vi "Write Previous State.vi"(8 "error in (no error)":errorcluster, 10 "Previous State":i32[](array[numeric]), 11 "FW Arduino Control in":refnum<class "FW Arduino Control.lvclass">) -> (0 "error out":errorcluster, 3 "FW Arduino Control out":refnum<class "FW Arduino Control.lvclass">)   [LabVIEW 2021, in "FW Arduino Control.lvclass"]
uses:
  FW Arduino Control.lvclass
  C:/Development/prime/Prime-RIMAS/Filter Wheel/Filter Wheel Object/Filter Wheel.lvclass
  Filter Wheel Object/Filter Wheel.lvclass
  FW Arduino Control.lvclass/FW Arduino Control.ctl
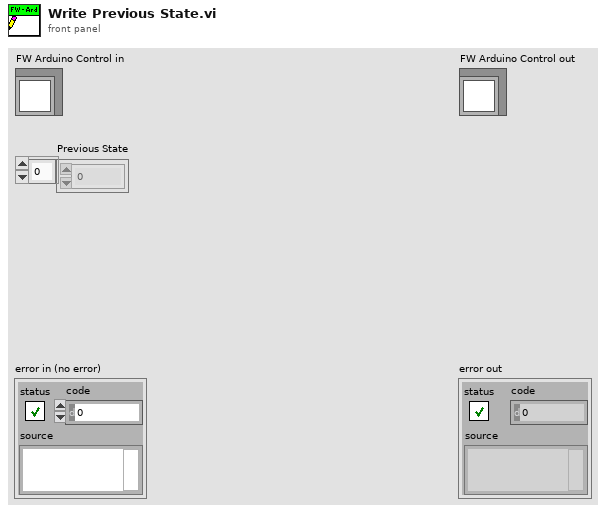
[diagram p1: front panel]
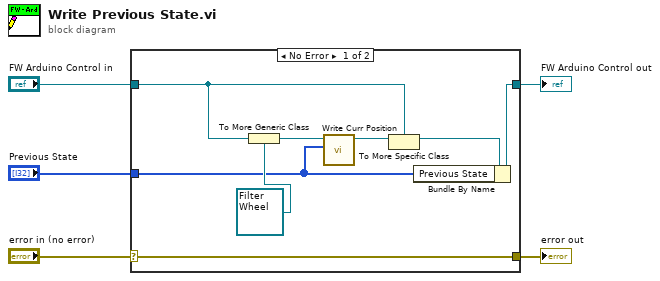
[diagram p0: block diagram]
diagram:
  n1 = case shown="No Error" "error in (no error)" {
    selector: "error in (no error)" -> [w13 w14]
    tunnel: [w13 w14] -> w4
    tunnel: [w12 w15] -> w2
    tunnel: "FW Arduino Control in" -> [w6 w15]
    tunnel: "Previous State" -> [w9 _]
    frame No Error {
      n2 = To More Generic Class(target class=refnum<class "Filter Wheel.lvclass"> refnum ("Filter Wheel.lvclass"), reference=w6) -> (generic class reference=w10:refnum<class "Filter Wheel.lvclass">)
      n3 = call-dynamic "Write Curr Position.vi"("Curr Position"=w9, "Filter Wheel in"=w10) -> ("Filter Wheel out"=w8:refnum<class "Filter Wheel.lvclass">)  [unwired: 8 in, 1 out]
      n4 = To More Specific Class(target class=w6, reference=w8) -> (specific class reference=w7:refnum<class "FW Arduino Control.lvclass">)  [unwired: 1 in, 1 out]
      n5 = Bundle By Name(cluster=w7, "Previous State"=w9) -> (w12:refnum<class "FW Arduino Control.lvclass">)
    }
    frame Error {
    }
  }
  "error out" <- w4
  "FW Arduino Control out" <- w2
